vi "POWER_SUPPLY_TEST.vi"() -> ()   [LabVIEW 2019]
panel:
  out "x+y":dbl
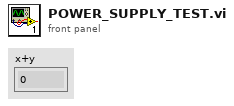
[diagram p1: front panel]
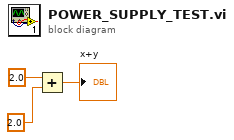
[diagram p0: block diagram]
diagram:
  n1 = Add(x=2.0, y=2.0) -> (x+y=→"x+y":dbl)
